vi "Read Target Processor.vi"(8 "error in (no error)":errorcluster, 11 "Node Ptr":T1 format="%.0x") -> (0 "error out":errorcluster, 2 "targetProcessor":i8 caption="Target Processor" min=-2 max=16 step=1, 3 "Node Ptr out":T1 format="%.0x")   [LabVIEW 2021, in "UDP-Custom-Device System Explorer.lvlib" / "Shared Packet Accessors.lvlib"]
uses:
  Shared Packet Accessors.lvlib
  <vilib>/NI VeriStand/Custom Device API/Custom Device Item Ref.ctl
  Shared/Constants.vi
  <vilib>/NI VeriStand/Custom Device API/Get Item Property (I32).vi
  <vilib>/NI VeriStand/Custom Device API/Custom Device API.lvlib
  Shared/UDP-Custom-Device Shared.lvlib
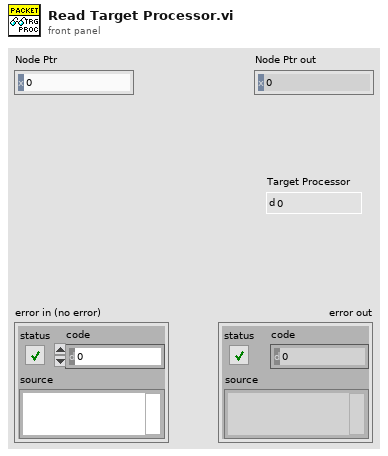
[diagram p1: front panel]
types:
  T1 = typedef "Custom Device API.lvlib/Custom Device Item Ref.ctl" = u64
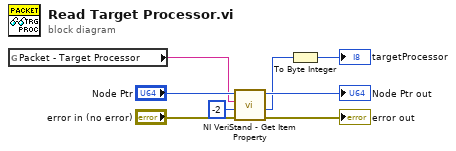
[diagram p0: block diagram]
diagram:
  n1 = global read "Constants.vi" "Packet - Target Processor"() -> (w4:string)
  n2 = call-poly <vilib>:"NI VeriStand - Get Item Property.vi"("error in (no error)"="error in (no error)", "Default Value"=-2, "Property Name"=w4, "Item Ref in"="Node Ptr") -> ("error out"=→"error out":errorcluster, "Value"=w2:i32, "Item Ref out"=→"Node Ptr out":T1)  [unwired: 4 in, 1 out]
  n3 = To Byte Integer(number=w2) -> (8bit integer=→"targetProcessor":i8)
